vi "TDC_recv_data.vi"(3 "时间数据":u32[](array[numeric])) -> (0 "粗计数":i32[](array[numeric]), 1 "b细计数":i32[](array[numeric]), 2 "a细计数":i32[](array[numeric]))   [LabVIEW 2014]
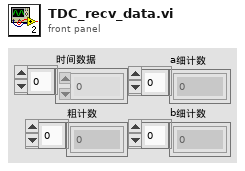
[diagram p1: front panel]
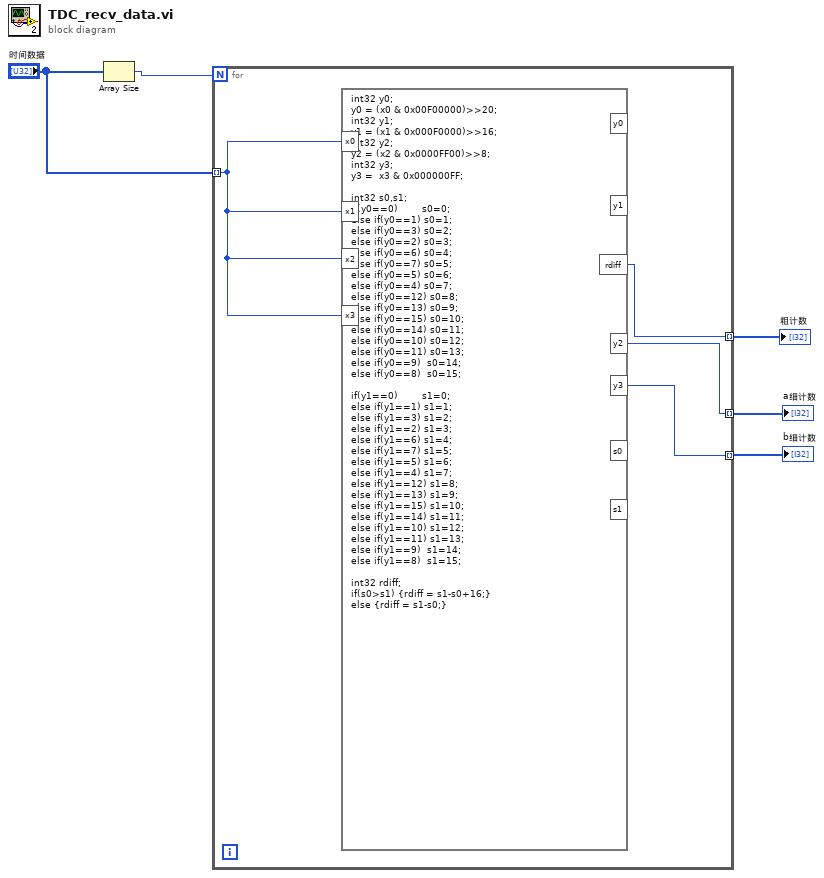
[diagram p0: block diagram]
diagram:
  n1 = Array Size(array="时间数据") -> (size(s)=w5:i32)
  n2 = for {
    N: w5 -> [_]
    tunnel: "时间数据" -> [w9] mode=indexing
    tunnel: [w8] -> w3 mode=indexing
    tunnel: [w7] -> w2 mode=indexing
    tunnel: [w6] -> w1 mode=indexing
    n3 = formula code="int32 y0;\ny0 = (x0 & 0x00F00000)>>20;\nint32 y1;\ny1 = (x1 & 0x000F0000)>>16;\nint32 y2;\ny2 = (x2 & 0x0000FF00)>>8;\nint32 y3;\ny3 =  x3 & 0x000000FF;\n\nint32 s0,s1;\nif(y0==0)        s0=0;\nelse if(y0==1) s0=1;\nelse if(y0==3) s0=2;\nelse if(y0==2) s0=3;\nelse if(y0==6) s0=4;\nelse if(y0==7) s0=5;\nelse if(y0==5) s0=6;\nelse if(y0==4) s0=7;\nelse if(y0==12) s0=8;\nelse if(y0==13) s0=9;\nelse if(y0==15) s0=10;\nelse if(y0==14) s0=11;\nelse if(y0==10) s0=12;\nelse if(y0==11) s0=13;\nelse if(y0==9)  s0=14;\nelse if(y0==8)  s0=15;\n\nif(y1==0)        s1=0;\nelse if(y1==1) s1=1;\nelse if(y1==3) s1=2;\nelse if(y1==2) s1=3;\nelse if(y1==6) s1=4;\nelse if(y1==7) s1=5;\nelse if(y1==5) s1=6;\nelse if(y1==4) s1=7;\nelse if(y1==12) s1=8;\nelse if(y1==13) s1=9;\nelse if(y1==15) s1=10;\nelse if(y1==14) s1=11;\nelse if(y1==10) s1=12;\nelse if(y1==11) s1=13;\nelse if(y1==9)  s1=14;\nelse if(y1==8)  s1=15;\n\nint32 rdiff;\nif(s0>s1) {rdiff = s1-s0+16;}\nelse {rdiff = s1-s0;}"("x1"=w9, "x2"=w9, "x3"=w9, "x0"=w9) -> ("y2"=w7:i32, "y3"=w6:i32, "rdiff"=w8:i32)  [unwired: 4 out]
  }
  "粗计数" <- w3
  "a细计数" <- w2
  "b细计数" <- w1
